vi "close.vi"(8 "error in (no error)":errorcluster) -> (0 "error out":errorcluster)   [LabVIEW 2013, in "TCP_IP.lvclass"]
uses:
  TCP_IP.lvclass
  TCP_IP.lvclass/TCP_IP.ctl
  Globals.vi
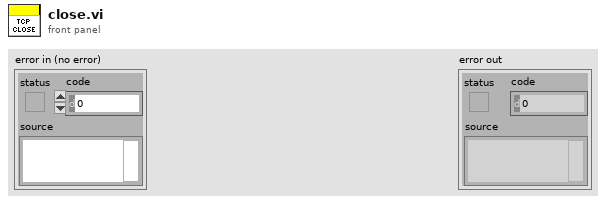
[diagram p1: front panel]
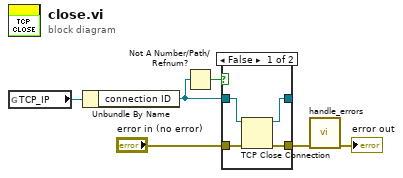
[diagram p0: block diagram]
diagram:
  n1 = global read "Globals.vi" "TCP_IP"() -> (w6:refnum<class "TCP_IP.lvclass">)
  n2 = Unbundle By Name(w6) -> ("connection ID"=w1:refnum<k5>)
  n3 = Not A Number/Path/Refnum?(number/path/refnum=w1) -> (NaN/Path/Refnum?=w4:bool)
  n4 = case shown="False" w4 {
    tunnel: [w10 w12] -> w3
    tunnel: w1 -> [w9 w11]
    tunnel: "error in (no error)" -> [w8 w12]
    tunnel: [w7 w11] -> _
    frame False {
      n5 = TCP Close Connection(connection ID=w9, error in (no error)=w8) -> (connection ID out=w7:refnum<k5>, error out=w10:errorcluster)  [unwired: 1 in]
    }
    frame True {
    }
  }
  n6 = call "handle_errors.vi"("error in (no error)"=w3) -> ("error out"=→"error out":errorcluster)  [unwired: 14 in]
